vi "Untitled 1.vi"() -> ()   [LabVIEW 2024]
uses:
  <vilib>/LabVIEW Open Source Project/Epoch Date & Time/epoch.UNIX/Epoch.UNIX.lvclass
panel:
  in  "Tab Control":enum32{"Page 1", "Page 2", "Page 3"}(tab)
  out "Waveform Chart":dbl(graph)
  out "output waveform":waveform(dbl)
  out "Waveform Chart 2":waveform(dbl)(graph)
  out "output waveform 2":waveform(dbl)
  out "Waveform Chart 3":waveform(dbl)(graph)
  out "output waveform 3":waveform(dbl)
  out "Waveform Chart 4":waveform(dbl)(graph)
  in  "stop":bool
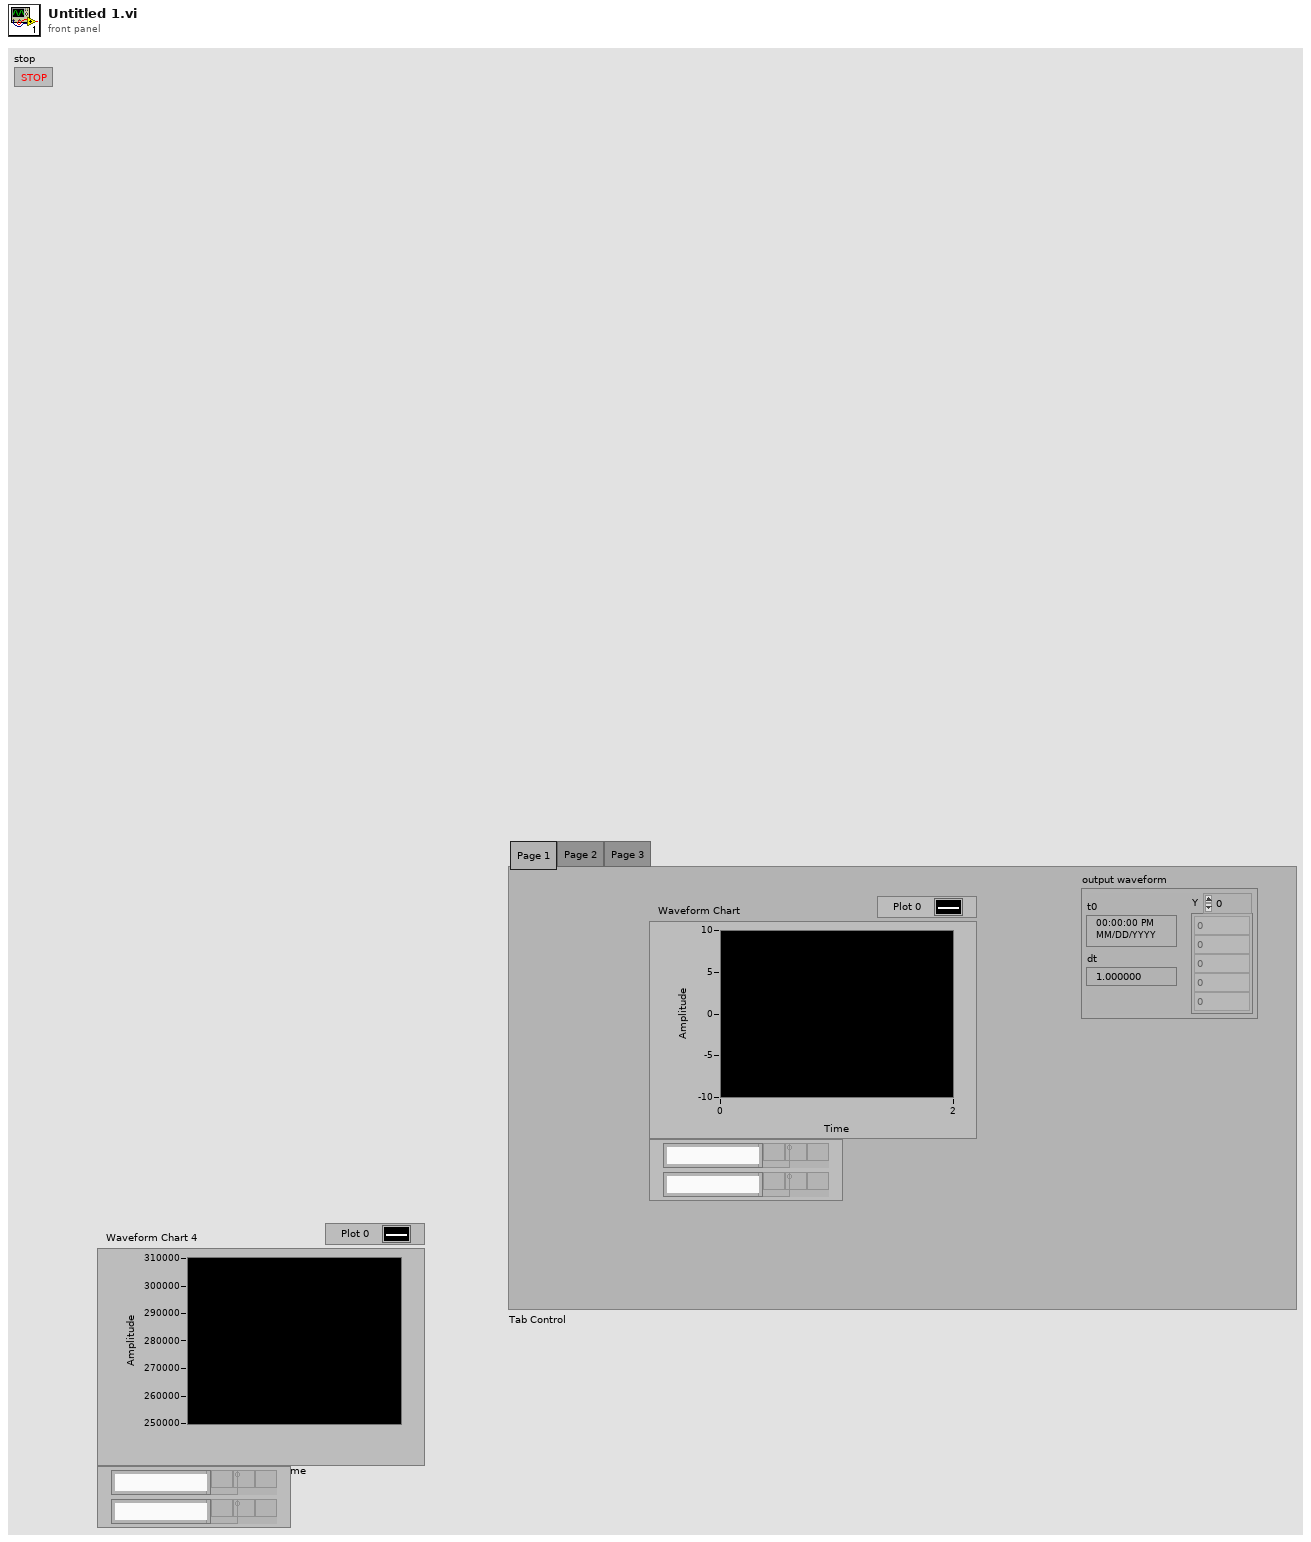
[diagram p1: front panel]
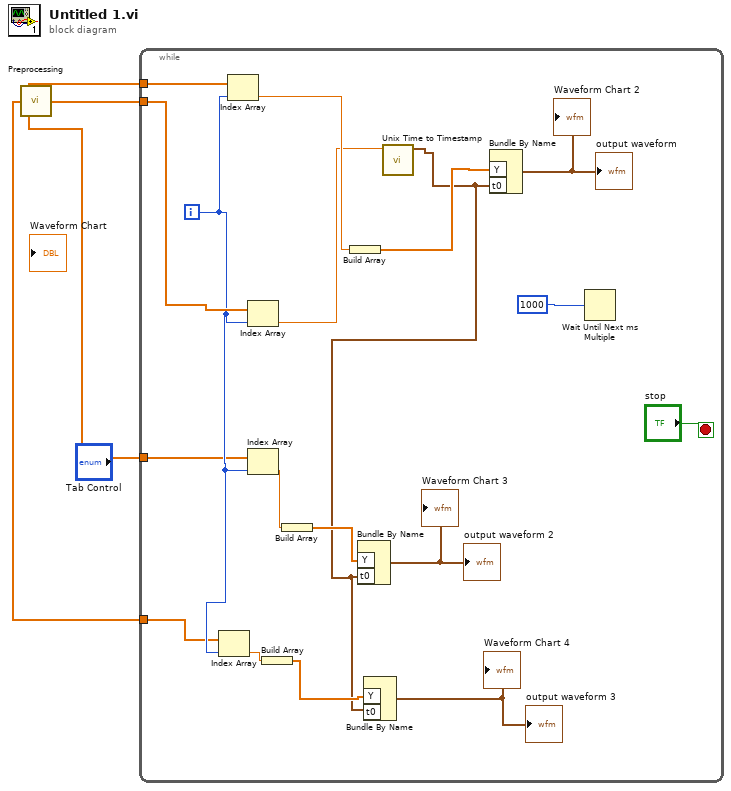
[diagram p0: block diagram]
diagram:
  n1 = call "Preprocessing.vi"() -> ("TimeStamp"=w4:dbl[], "Potência Ativa A 3"=w2:dbl[], "Potência Ativa A 2"=w1:dbl[], "Potência Ativa A"=w3:dbl[])
  n2 = while {
    tunnel: w4 -> [w22]
    tunnel: w3 -> [w21]
    tunnel: w2 -> [w7]
    tunnel: w1 -> [w6]
    i -> [w8]
    stop <- "stop" stop-if-true
    n3 = Index Array(array=w6, index=w8) -> (element=w9:dbl)
    n4 = Index Array(array=w21, index=w8) -> (element=w17:dbl)
    n5 = Index Array(array=w22, index=w8) -> (element=w16:dbl)
    n6 = Index Array(array=w7, index=w8) -> (element=w13:dbl)
    n7 = Build Array(w9) -> (w10:dbl[])
    n8 = Build Array(w13) -> (w14:dbl[])
    n9 = Build Array(w17) -> (w20:dbl[])
    n10 = call <vilib>:"Unix Time to Timestamp.vi"("Unix Time (s)"=w16) -> ("Timestamp"=w5:timestamp)  [unwired: 9 in, 1 out]
    n11 = Bundle By Name("Y"=w14, "t0"=w5) -> (→"output waveform 2" →"Waveform Chart 3":waveform(dbl))  [unwired: 1 in]
    n12 = Bundle By Name("Y"=w10, "t0"=w5) -> (→"output waveform 3" →"Waveform Chart 4":waveform(dbl))  [unwired: 1 in]
    n13 = Bundle By Name("Y"=w20, "t0"=w5) -> (→"output waveform" →"Waveform Chart 2":waveform(dbl))  [unwired: 1 in]
    n14 = Wait Until Next ms Multiple(millisecond multiple=u32 1000) -> ()  [unwired: 1 out]
  }
